vi "Mathcad_App_Open.vi"(7 "Visible":bool=TRUE, 8 "error in (no error)":errorcluster) -> (0 "error out (no error)":errorcluster, 3 "Mathcad.IMathcadApplication":refnum<k7>)   [LabVIEW 2015]
doc: "Opens a Mathcad Application. If this is the second call to this VI then it re-retrieves the Mathcad Application Reference that was already opened and sets the Application Reference to Visible or not Visible based in the input, \"Visible\". If the Mathcad Application reference has been lost or has been closed then it opens a new reference. If this VI is re-retrieveing a Mathcad Application Reference and fails to set the property to visible or not visible, it will open a new Mathcad Application Reference. Opening a new reference will typically take several seconds while re-retrieving an open reference only takes a few miliseconds.\n\nInputs\nVisible - If true then the Mathcad Application User Interface is visible.\n\nOutputs\nMathcad Application Reference- Reference to the Mathcad Application Class"
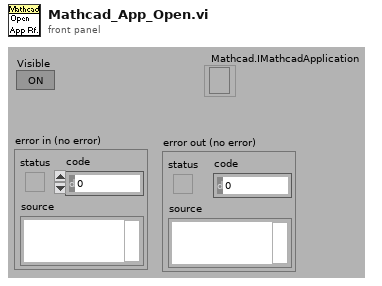
[diagram p1: front panel]
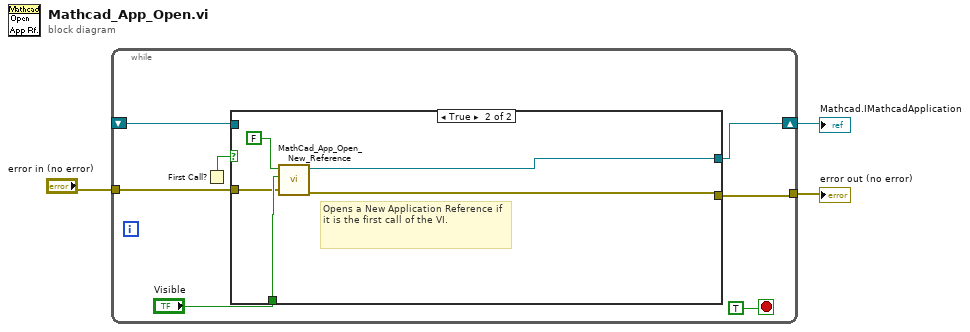
[diagram p0: block diagram]
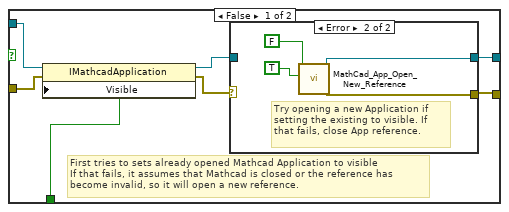
[diagram p2: hidden frame]
diagram:
  n1 = while {
    shift-right: [w5] -> w1
    shift-left: _ -> [w8]
    tunnel: [w4] -> w3
    tunnel: "error in (no error)" -> [w6]
    stop <- TRUE stop-if-true
    n2 = First Call?() -> (First Call?: T/F=w9:bool)
    n3 = case shown="True" w9 {
      tunnel: [w13 w27] -> w5
      tunnel: w8 -> [w17 _]
      tunnel: "Visible" -> [w16 w26]
      tunnel: [w12 w25] -> w4
      tunnel: w6 -> [w15 w24]
      frame False {
        # "First tries to sets already opened Mathcad Application to visible\nIf that fails, it assumes that Mathcad is closed or the reference has become invalid, so it will open a new reference."
        n4 = property class="IMathcadApplication"(reference=w17, error in=w15, "Visible"=w16) -> (reference out=w11:refnum<k7>, error out=w14:errorcluster)
        n5 = case shown="Error" w14 {
          selector: w14 -> [w19 _]
          tunnel: [w18 w21] -> w13
          tunnel: [w19 w20] -> w12
          tunnel: w11 -> [w18 _]
          frame No Error {
          }
          frame Error {
            # "Try opening a new Application if \nsetting the existing to visible. If\nthat fails, close App reference."
            n6 = call "MathCad_App_Open_New_Reference.vi"("Visible"=TRUE, "open new instance"=FALSE) -> ("error out (no error)"=w20:errorcluster, "IMathcadApp Ref"=w21:refnum<k7>)  [unwired: 8 in]
          }
        }
      }
      frame True {
        # "Opens a New Application Reference if it is the first call of the VI."
        n7 = call "MathCad_App_Open_New_Reference.vi"("error in (no error)"=w24, "Visible"=w26, "open new instance"=FALSE) -> ("error out (no error)"=w25:errorcluster, "IMathcadApp Ref"=w27:refnum<k7>)  [unwired: 7 in]
      }
    }
  }
  "error out (no error)" <- w3
  "Mathcad.IMathcadApplication" <- w1
